vi "Length-delimited Decoder.vi"(7 "Optional":bool, 8 "error in (no error)":errorcluster, 9 "Array":u8[](array[numeric]) format="%02x", 10 "Key":i32=-1) -> (0 "error out":errorcluster, 1 "array w/ subset deleted":u8[](array[numeric]), 2 "Read Key":i32, 3 "Length-delimited":u8[](array[numeric]))   [LabVIEW 2017]
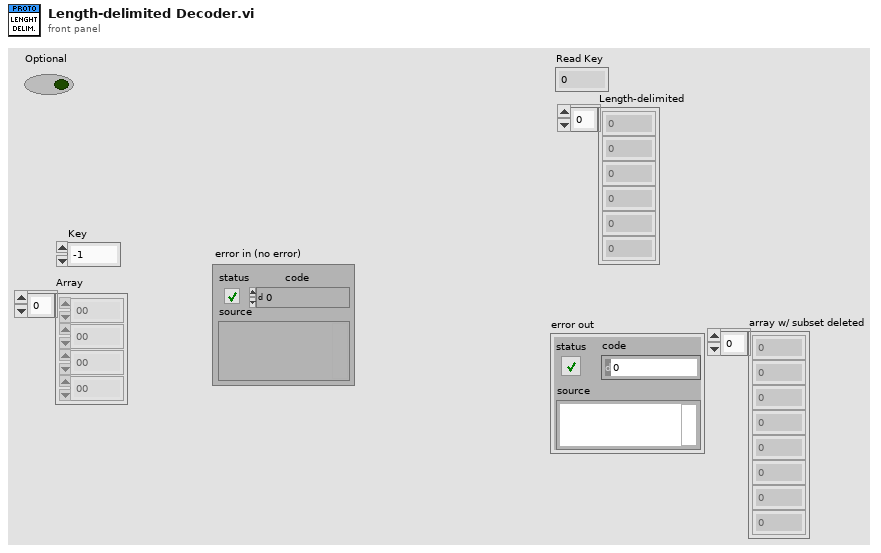
[diagram p1: front panel]
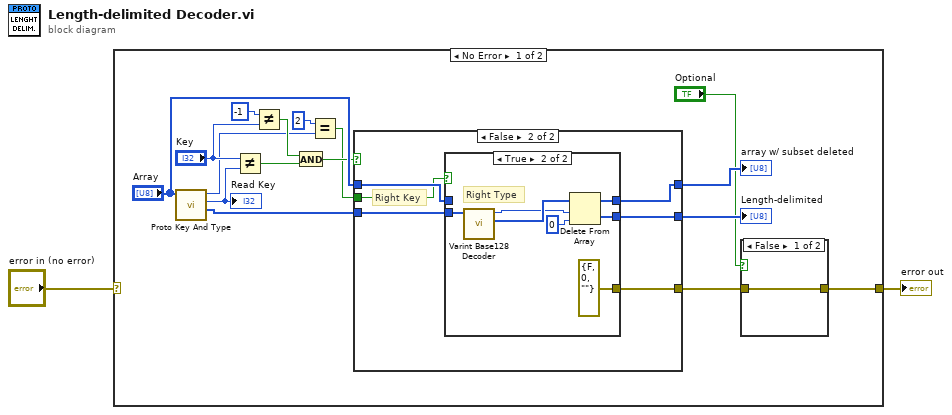
[diagram p0: block diagram]
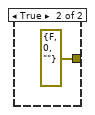
[diagram p2: hidden frame]
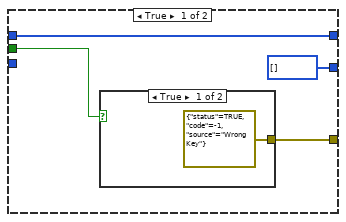
[diagram p3: hidden frame]
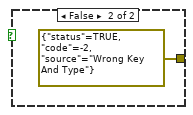
[diagram p4: hidden frame]
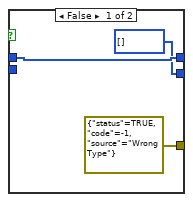
[diagram p5: hidden frame]
diagram:
  n1 = case shown="No Error" "error in (no error)" {
    selector: "error in (no error)" -> [_ w43]
    tunnel: [w3 w43] -> w1
    frame No Error {
      n2 = call "Proto Key And Type.vi"("Array"="Array") -> ("array w/ subset deleted"=w18:u8[], "Key"=w7:i32, "Type"=w10:i32)  [unwired: 8 in]
      "Read Key" <- w7
      n3 = Not Equal?(x="Key", y=w7) -> (x != y?=w13:bool)
      n4 = Not Equal?(x=-1, y="Key") -> (x != y?=w15:bool)
      n5 = And(x=w15, y=w13) -> (x .and. y?=w12:bool)
      n6 = Equal?(x=2, y=w10) -> (x = y?=w9:bool)
      n7 = case shown="False" w12 {
        tunnel: w18 -> [_ w32]
        tunnel: "Array" -> [w22 w31]
        tunnel: w9 -> [w24 w30]
        tunnel: [w23 w29] -> w4
        tunnel: [w22 w28] -> w8
        tunnel: [u8[] [] ("array w/ subset deleted") w27] -> w6
        frame True {
          n8 = case shown="True" w24 {
            tunnel: [errorcluster {"status"=TRUE, "code"=-1, "source"="Wrong Key"} ("error in (no error)") errorcluster {"status"=TRUE, "code"=-2, "source"="Wrong Key And Type"} ("error in (no error)")] -> w23
            frame True {
            }
            frame False {
            }
          }
        }
        frame False {
          # "Right Key"
          n9 = case shown="True" w30 {
            tunnel: [errorcluster {"status"=TRUE, "code"=-1, "source"="Wrong Type"} ("error in (no error)") errorcluster {"status"=FALSE, "code"=0, "source"=""} ("error in (no error)")] -> w29
            tunnel: w32 -> [_ w41]
            tunnel: [w34 w37] -> w28
            tunnel: w31 -> [w34 _]
            tunnel: [u8[] [] ("array w/ subset deleted") w36] -> w27
            frame False {
            }
            frame True {
              # "Right Type"
              n10 = call "Varint Base128 Decoder.vi"("Array"=w41) -> ("array w/ subset deleted"=w40:u8[], "Numeric"=w39:i32)  [unwired: 9 in]
              n11 = Delete From Array(array=w40, length=w39, index=0) -> (deleted portion=w36:u8[], array with subset deleted=w37:u8[])
            }
          }
        }
      }
      "array w/ subset deleted" <- w8
      "Length-delimited" <- w6
      n12 = case shown="False" "Optional" {
        tunnel: w4 -> [w19 _]
        tunnel: [w19 errorcluster {"status"=FALSE, "code"=0, "source"=""} ("error in (no error)")] -> w3
        frame False {
        }
        frame True {
        }
      }
    }
    frame Error {
    }
  }
  "error out" <- w1
